vi "readDCMeasurement.vi"(0 "NInstrSim":refnum<class "NInstrSim.lvclass">, 5 "error in (no error)":errorcluster) -> (14 "dup NInstrSim":refnum<class "NInstrSim.lvclass">, 16 "DC Measurement":dbl format="%_6g", 19 "error out":errorcluster)   [LabVIEW 2009, in "HB_Device_Examples.lvlib" / "NInstrSim.lvclass"]
doc: "Reads a DC measurement from the NI Instrument Simulator."
uses:
  NInstrSim.lvclass
  NInstrSim.lvclass/NInstrSim.ctl
  lib.lib/HGF_LVC/HGF_BaseClasses/HGF_TriggeredEvent/HGF_TriggeredEvent.lvclass
  lib.lib/HGF_LVC/HGF_DeviceBaseClasses/HGF_VISADevice/HGF_VISADevice.lvclass
  non_GPL/instr.lib/NI Instrument Simulator/NI Instrument Simulator.lvlib
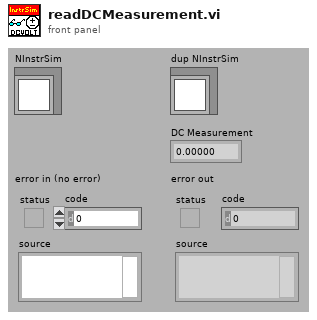
[diagram p1: front panel]
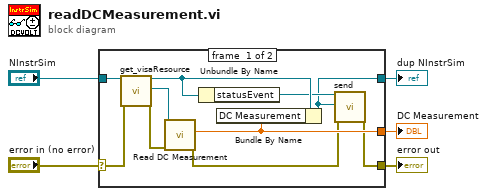
[diagram p0: block diagram]
diagram:
  n1 = case shown="No Error" "error in (no error)" {
    selector: "error in (no error)" -> [w12 w17]
    tunnel: [w6 w17] -> w4
    tunnel: [w8 w16] -> w2
    tunnel: "NInstrSim" -> [w15 w16]
    tunnel: [w11 _] -> w1
    frame #0 {
      n2 = call "get_visaResource.vi"("HGF_VISADevice"=w15, "error in (no error)"=w12) -> ("dup HGF_VISADevice"=w10:refnum<class "NInstrSim.lvclass">, "VISA Resource Name"=w14:refnum<visa-resource-name>, "error out"=w13:errorcluster)  [unwired: 15 out]
      n3 = call "Read DC Measurement.vi"("error in (no error)"=w13, "VISA resource name"=w14) -> ("error out"=w7:errorcluster, "DC Measurement"=w11:dbl)  [unwired: 8 out]
      n4 = Unbundle By Name(w10) -> ("statusEvent"=w9:refnum<class "HGF_TriggeredEvent.lvclass">)
      n5 = Bundle By Name(cluster=w10, "DC Measurement"=w11) -> (w8:refnum<class "NInstrSim.lvclass">)
      n6 = call-dynamic "send.vi"("HGF_Event"=w9, "Object"=w8, "error in (no error)"=w7) -> ("error out"=w6:errorcluster)  [unwired: 2 in, 14 out]
    }
    frame #1 {
    }
  }
  "error out" <- w4
  "dup NInstrSim" <- w2
  "DC Measurement" <- w1
